vi "Is a DQMH Module.vi"(8 "error in":errorcluster, 11 "Library":refnum<vi>) -> (0 "error out":errorcluster, 1 "Cloneable?":bool, 2 "Is DQMH?":bool, 3 "Library Refnum":refnum<vi>)   [LabVIEW 2020, in "DQMH_API.lvlib"]
uses:
  DQMH_API.lvlib
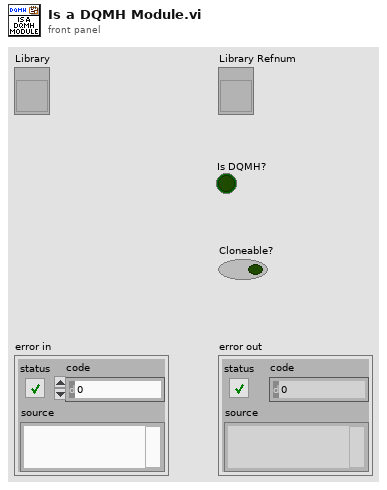
[diagram p1: front panel]
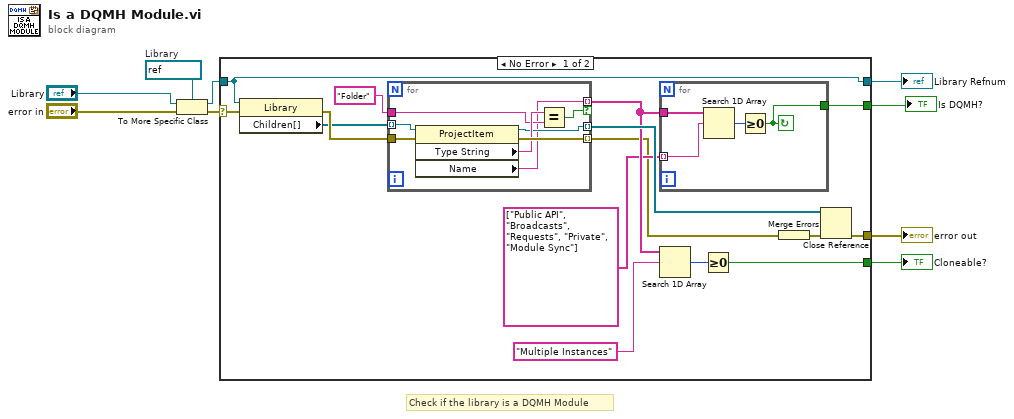
[diagram p0: block diagram]
diagram:
  w6 = refnum<vi> refnum  # Library
  # "Check if the library is a DQMH Module"
  n1 = To More Specific Class(target class=w6, reference="Library", error in="error in") -> (specific class reference=w5:refnum<vi>, error out=w8:errorcluster)
  n2 = case shown="No Error" w8 {
    selector: w8 -> [w24 _]
    tunnel: w5 -> [w19 _]
    tunnel: [w20 _] -> w1
    tunnel: [w19 _] -> w2
    tunnel: [w23 _] -> w7
    tunnel: [w18 _] -> w3
    frame No Error {
      n3 = property class="Library"(reference=w19, error in=w24) -> (error out=w22:errorcluster, "Children[]"=w16:refnum<vi>[])  [unwired: 1 out]
      n4 = for {
        tunnel: [w29] -> w12 mode=indexing if=w30
        tunnel: w22 -> [w36]
        tunnel: [w35] -> w10 mode=indexing
        tunnel: [w32] -> w15 mode=indexing
        tunnel: w16 -> [w34] mode=indexing
        tunnel: "Folder" ("Type") -> [w31]
        n5 = property class="ProjectItem"(reference=w34, error in=w36) -> (reference out=w32:refnum<vi>, error out=w35:errorcluster, "Type String"=w33:string, "Name"=w29:string)
        n6 = Equal?(x=w33, y=w31) -> (x = y?=w30:bool)
      }
      n7 = for {
        tunnel: string[] ["Public API", "Broadcasts", "Requests", "Private", "Module Sync"] -> [w28] mode=indexing
        tunnel: w12 -> [w27]
        tunnel: [w25] -> w20
        stop <- w25 continue-if-true
        n8 = Search 1D Array(1D array=w27, element=w28) -> (index of element=w26:i32)  [unwired: 1 in]
        n9 = Greater Or Equal To 0?(x=w26) -> (x >= 0?=w25:bool)
      }
      n10 = Search 1D Array(1D array=w12, element="Multiple Instances") -> (index of element=w14:i32)  [unwired: 1 in]
      n11 = Greater Or Equal To 0?(x=w14) -> (x >= 0?=w18:bool)
      n12 = Merge Errors(w10) -> (w21:errorcluster)
      n13 = Close Reference(reference=w15, error in (no error)=w21) -> (error out=w23:errorcluster)
    }
    frame Error {
    }
  }
  "Cloneable?" <- w3
  "Library Refnum" <- w2
  "error out" <- w7
  "Is DQMH?" <- w1
